vi "Error Handler.vi"(7 "Error Handler States":T1(ring), 8 "Error In":errorcluster) -> (0 "Error Out":errorcluster)   [LabVIEW 2012, in "OpenCLV x64.lvlib"]
uses:
  OpenCLV x64.lvlib
  Error Control.ctl
panel:
  in  "Stop Button":bool
  in  "Tree":string(tree)
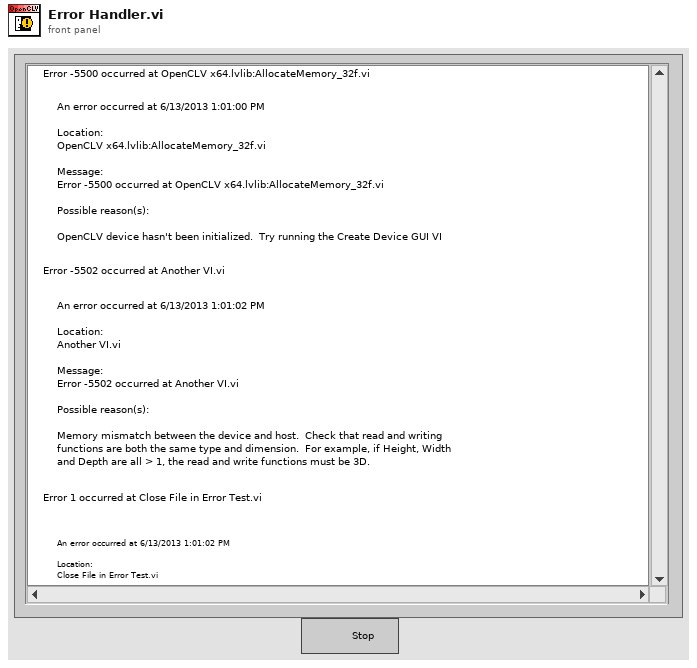
[diagram p1: front panel]
types:
  T1 = enum16{"Initialize", "Add Error", "View Error Log", "Save Error Log", "Set Verbose Mode", "Set Quite Mode"}
  T2 = typedef "OpenCLV x64.lvlib/Error Control.ctl" = cluster{"Error In":errorcluster, "Date / Time of Error":string}
  T3 = enum32{"Invalid", "Standard", "Closed", "Hidden", "Minimized", "Maximized"}
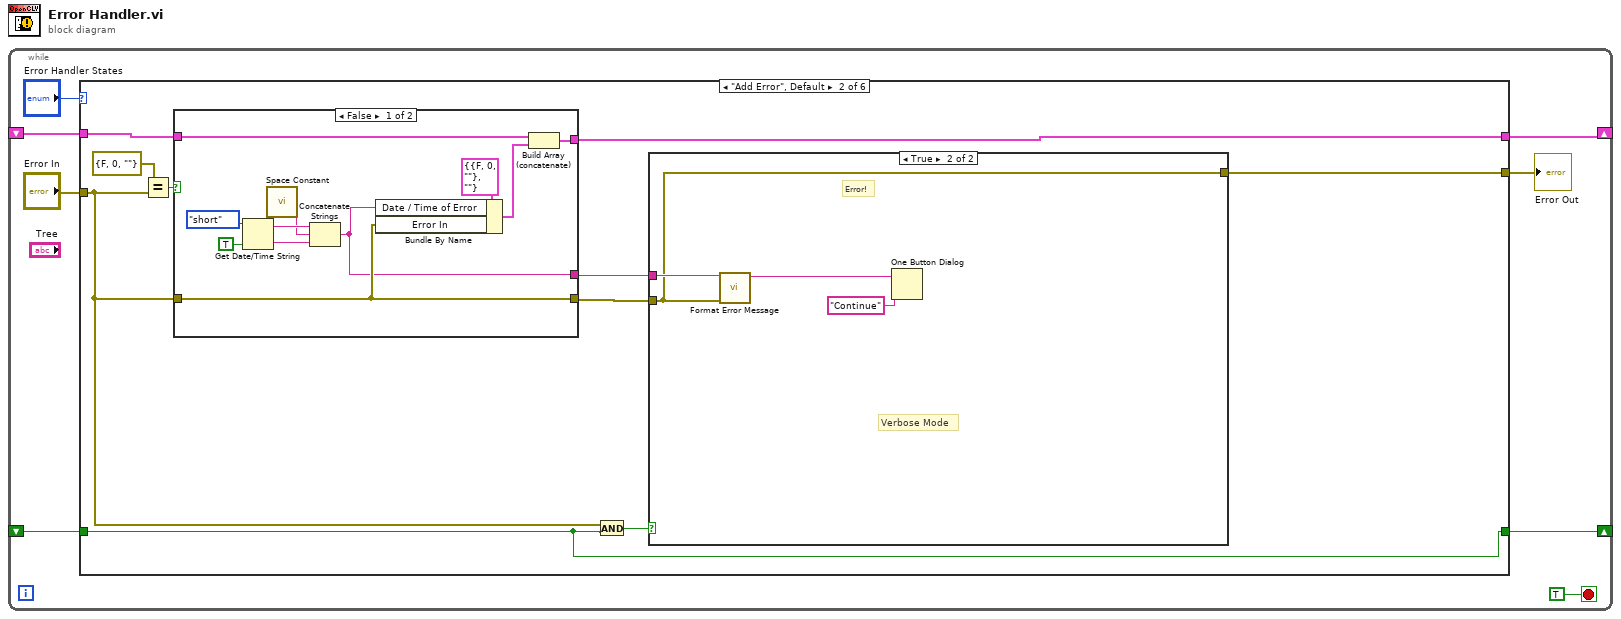
[diagram p0: block diagram]
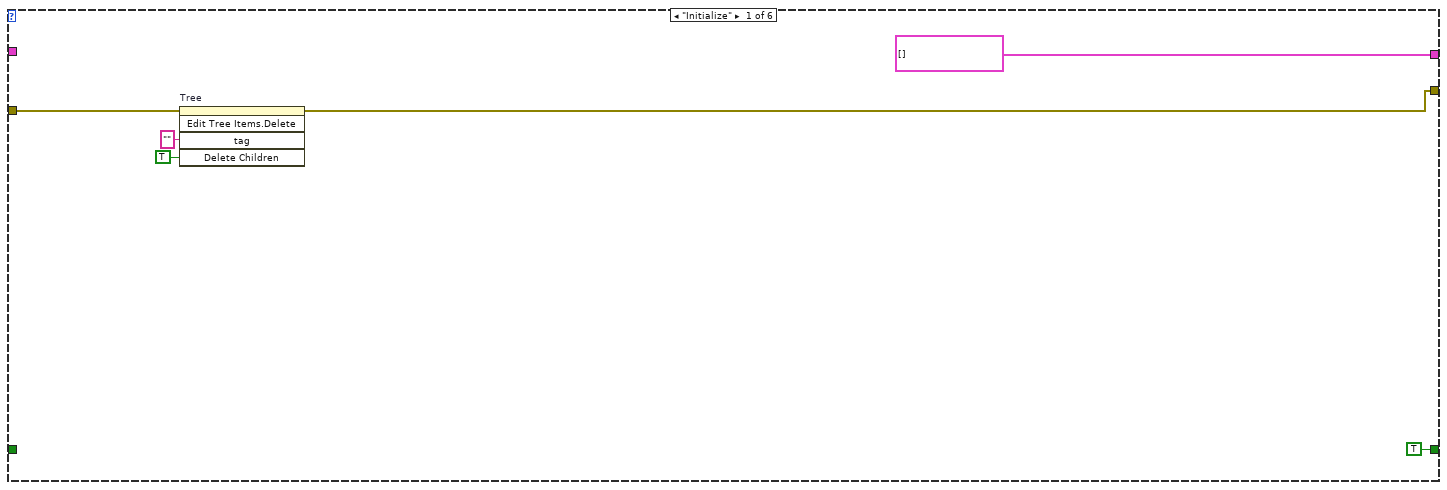
[diagram p2: hidden frame]
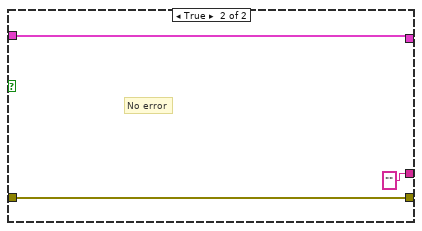
[diagram p4: hidden frame]
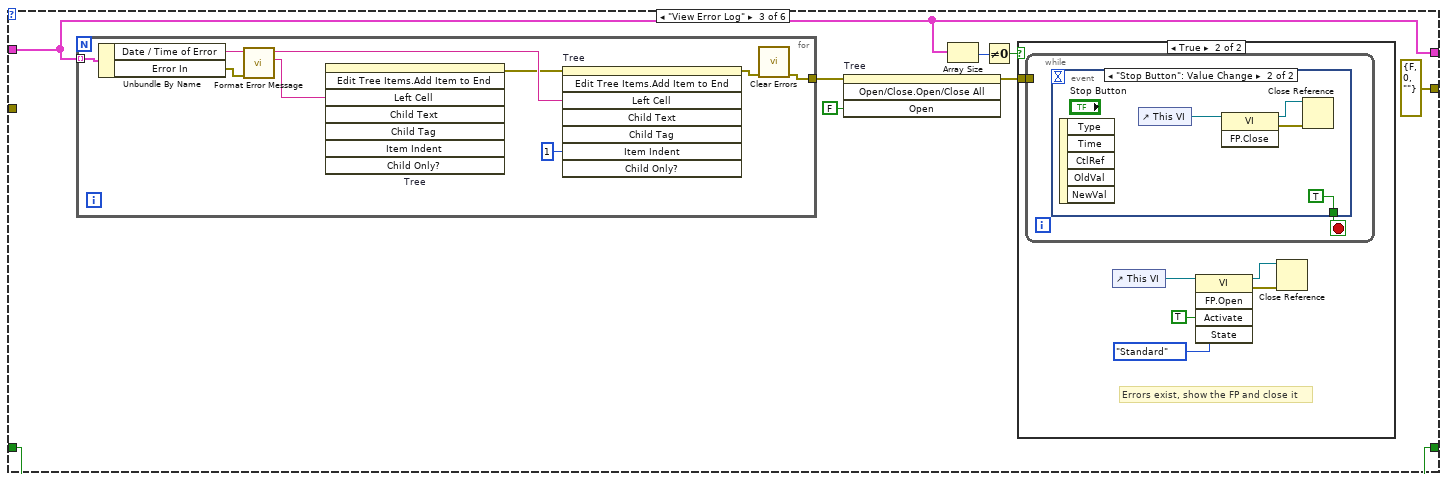
[diagram p5: hidden frame]
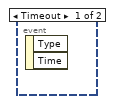
[diagram p7: hidden frame]
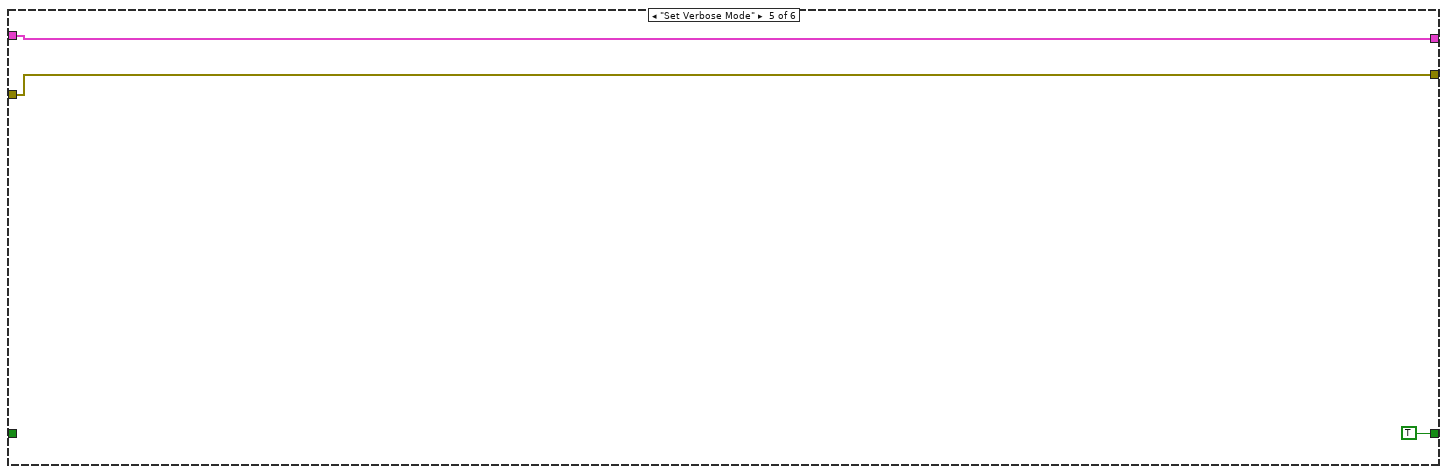
[diagram p9: hidden frame]
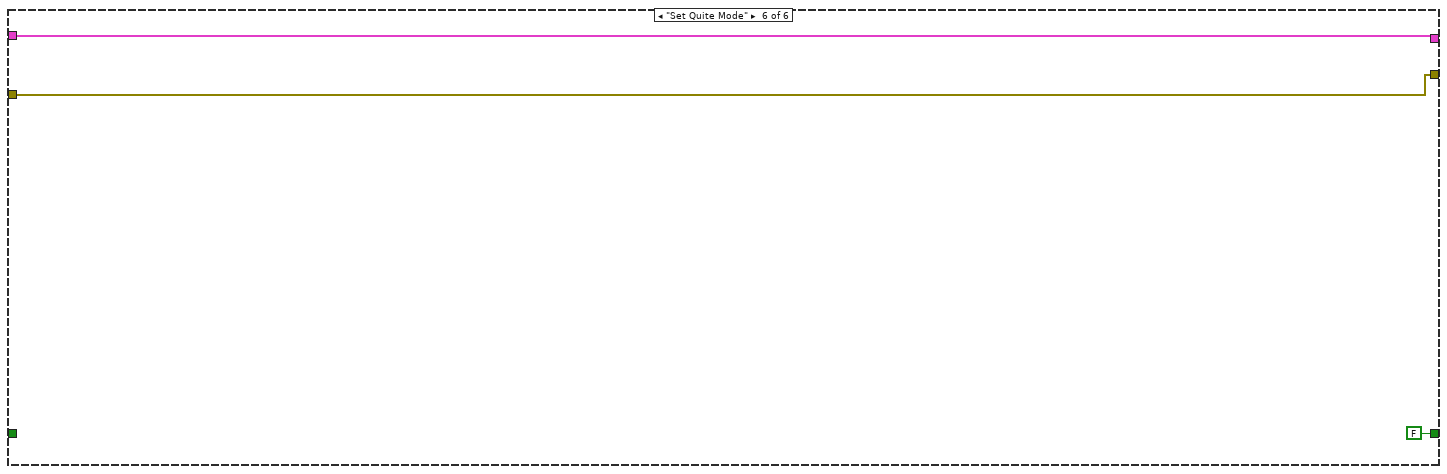
[diagram p10: hidden frame]
diagram:
  n1 = while {
    shift-right: [w4] -> _
    shift-left: _ -> [w5]
    shift-right: [w2] -> _
    shift-left: _ -> [w1]
    stop <- TRUE stop-if-true
    n2 = case shown="\"Add Error\", Default" "Error Handler States" {
      tunnel: "Error In" -> [w10 w15 _ w74 w76 w78]
      tunnel: w5 -> [_ w23 w44 w73 w75 w79]
      tunnel: [T2[] [] ("Array") w22 w44 w73 w75 w79] -> w4
      tunnel: [w13 w18 errorcluster {"status"=FALSE, "code"=0, "source"=""} ("Error In") w74 w76 w78] -> w3
      tunnel: [TRUE w16 w50 w72 TRUE FALSE] -> w2
      tunnel: w1 -> [_ w16 w50 w72 _ _]
      frame "Initialize" {
        n3 = invoke on="Tree" class="Tree (strict)" method="Edit Tree Items.Delete"(error in=w10, "tag"="" ("Tag"), "Delete Children"=TRUE ("Delete Children?")) -> (error out=w13:errorcluster)  [unwired: 2 in, 4 out]
      }
      frame "Add Error", Default {
        n4 = Equal?(x=errorcluster {"status"=FALSE, "code"=0, "source"=""} ("y"), y=w15) -> (x = y?=w24:bool)
        n5 = case shown="False" w24 {
          tunnel: w23 -> [w33 w43]
          tunnel: [w32 w43] -> w22
          tunnel: [w31 w42] -> w20
          tunnel: w15 -> [w31 w42]
          tunnel: [w30 ""] -> w19
          frame False {
            n6 = Get Date/Time String(date format (0)=enum16{"short", "long", "abbreviated"}."short", want seconds? (F)=TRUE) -> (date string=w38:string, time string=w39:string)  [unwired: 1 in]
            n7 = call <vilib>:"Space Constant.vi"() -> ("String"=w37:string)
            n8 = Concatenate Strings(w38, w37, w39) -> (w30:string)
            n9 = Bundle By Name(cluster=T2 {"Error In"={"status"=FALSE, "code"=0, "source"=""}, "Date / Time of Error"=""} ("Error Control"), "Date / Time of Error"=w30, "Error In"=w31) -> (w34:T2)
            n10 = Build Array (concatenate)(w33, w34) -> (w32:T2[])
          }
          frame True {
            # "No error"
          }
        }
        n11 = And(x=w15, y=w16) -> (x .and. y?=w17:bool)
        n12 = case shown="True" w17 {
          tunnel: w20 -> [w25 w28]
          tunnel: w19 -> [_ w29]
          tunnel: [w25 w28] -> w18
          frame False {
            # "Quite Mode"
          }
          frame True {
            # "Verbose Mode"
            # "Error!"
            n13 = call "Format Error Message.vi"("error in (no error)"=w28, "Date / Time"=w29) -> ("Error Message"=w26:string)  [unwired: 8 in, 1 out]
            n14 = One Button Dialog(message=w26, button name ("OK")="Continue" ("F button name (\"Cancel\")")) -> ()  [unwired: 1 out]
          }
        }
      }
      frame "View Error Log" {
        n15 = for {
          tunnel: w44 -> [w71] mode=indexing
          tunnel: [w63] -> w49
          n16 = Unbundle By Name(w71) -> ("Date / Time of Error"=w69:string, "Error In"=w70:errorcluster)
          n17 = call "Format Error Message.vi"("error in (no error)"=w70, "Date / Time"=w69) -> ("Error Substring"=w66:string, "Error Message"=w67:string)  [unwired: 8 in]
          n18 = invoke on="Tree" class="Tree (strict)" method="Edit Tree Items.Add Item to End"("Left Cell"=w66) -> (error out=w65:errorcluster)  [unwired: 7 in, 7 out]
          n19 = invoke on="Tree" class="Tree (strict)" method="Edit Tree Items.Add Item to End"(error in=w65, "Left Cell"=w67, "Item Indent"=1 ("New Item Indentation")) -> (error out=w64:errorcluster)  [unwired: 5 in, 7 out]
          n20 = call <vilib>:"Clear Errors.vi"("error in (no error)"=w64) -> ("error out"=w63:errorcluster)  [unwired: 6 in]
        }
        n21 = invoke on="Tree" class="Tree (strict)" method="Open/Close.Open/Close All"(error in=w49, "Open"=FALSE ("Open?")) -> (error out=w47:errorcluster)  [unwired: 2 in, 3 out]
        n22 = Array Size(array=w44) -> (size(s)=w45:i32)
        n23 = Not Equal To 0?(x=w45) -> (x != 0?=w46:bool)
        n24 = case shown="True" w46 {
          tunnel: w47 -> [_ w52]
          frame False {
            # "No errors, don't show this VI"
          }
          frame True {
            # "Errors exist, show the FP and close it"
            n25 = while {
              tunnel: w52 -> [_]
              stop <- w58 stop-if-true
              n26 = event shown="[1] \"Stop Button\": Value Change" {
                selector: _ -> [_ _]
                dyn-events: _ -> [_ _]
                timeout: _ -> [_ _]
                tunnel: [_ TRUE] -> w58
                event Timeout {
                  n27 = event-data() -> ()  [unwired: 1 in, 2 out]
                }
                event "Stop Button": Value Change {
                  n28 = event-data() -> ()  [unwired: 1 in, 5 out]
                  n29 = control-ref of="This VI"() -> (w59:refnum<vi>)
                  n30 = invoke class="VI" method="FP.Close"(reference=w59) -> (reference out=w61:refnum<vi>, error out=w60:errorcluster)  [unwired: 2 in, 1 out]
                  n31 = Close Reference(reference=w61, error in (no error)=w60) -> ()  [unwired: 1 out]
                }
              }
            }
            n32 = control-ref of="This VI"() -> (w57:refnum<vi>)
            n33 = invoke class="VI" method="FP.Open"(reference=w57, "Activate"=TRUE ("Activate?"), "State"=T3."Standard") -> (reference out=w53:refnum<vi>, error out=w54:errorcluster)  [unwired: 2 in, 3 out]
            n34 = Close Reference(reference=w53, error in (no error)=w54) -> ()  [unwired: 1 out]
          }
        }
      }
      frame "Save Error Log" {
      }
      frame "Set Verbose Mode" {
      }
      frame "Set Quite Mode" {
      }
    }
    "Error Out" <- w3
  }
